vi "Read UI References.vi"(8 "error in (no error)":errorcluster, 11 "UI Console in":refnum<class "UI Console.lvclass">) -> (0 "error out":errorcluster, 2 "UI References":T1, 3 "UI Console out":refnum<class "UI Console.lvclass">)   [LabVIEW 2019, in "UI Console.lvclass"]
uses:
  UI Console.lvclass
  TypeDef/UI References.ctl
  UI Console.lvclass/UI Console.ctl
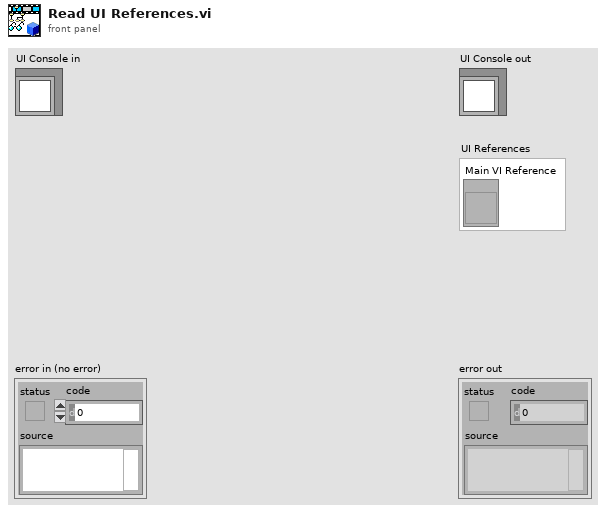
[diagram p1: front panel]
types:
  T1 = typedef "UI References.ctl" = cluster{"Main VI Reference":refnum<vi>}
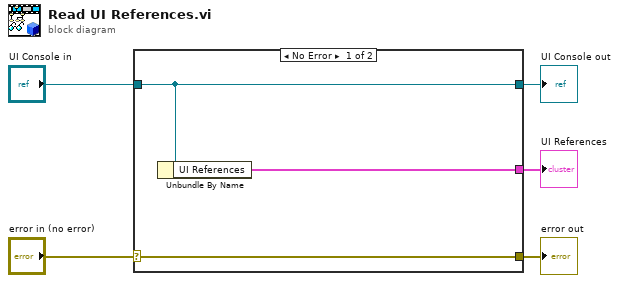
[diagram p0: block diagram]
diagram:
  n1 = case shown="No Error" "error in (no error)" {
    selector: "error in (no error)" -> [w8 w9]
    tunnel: [w8 w9] -> w4
    tunnel: [w7 w10] -> w2
    tunnel: "UI Console in" -> [w7 w10]
    tunnel: [w6 _] -> w1
    frame No Error {
      n2 = Unbundle By Name(w7) -> ("UI References"=w6:T1)
    }
    frame Error {
    }
  }
  "error out" <- w4
  "UI Console out" <- w2
  "UI References" <- w1
